vi "Open.vi"(8 "error in (no error)":errorcluster, 10 "Create if not exists? (T)":bool=TRUE, 11 "Path":path) -> (0 "error out":errorcluster, 1 "File Exists?":bool, 2 "File Created?":bool, 3 "LabVIEW-Config.lvlib:LabVIEW-Config.lvclass":refnum<class "LabVIEW-Config.lvclass">)   [LabVIEW 2017, in "LabVIEW-Config.lvlib" / "LabVIEW-Config.lvclass"]
uses:
  LabVIEW-Config.lvclass
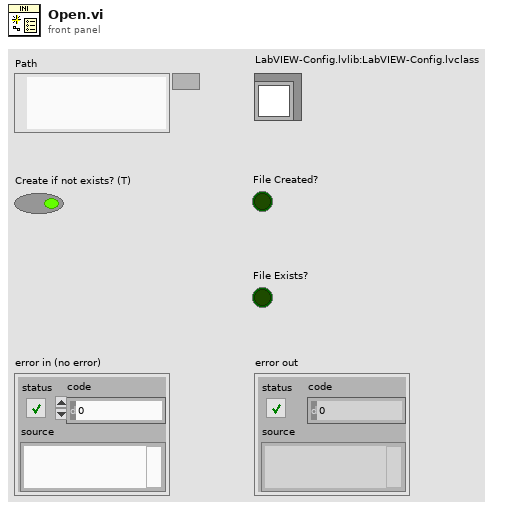
[diagram p1: front panel]
types:
  T1 = enum16{"open", "replace", "create", "open or create", "replace or create", "replace or create with confirmation"}
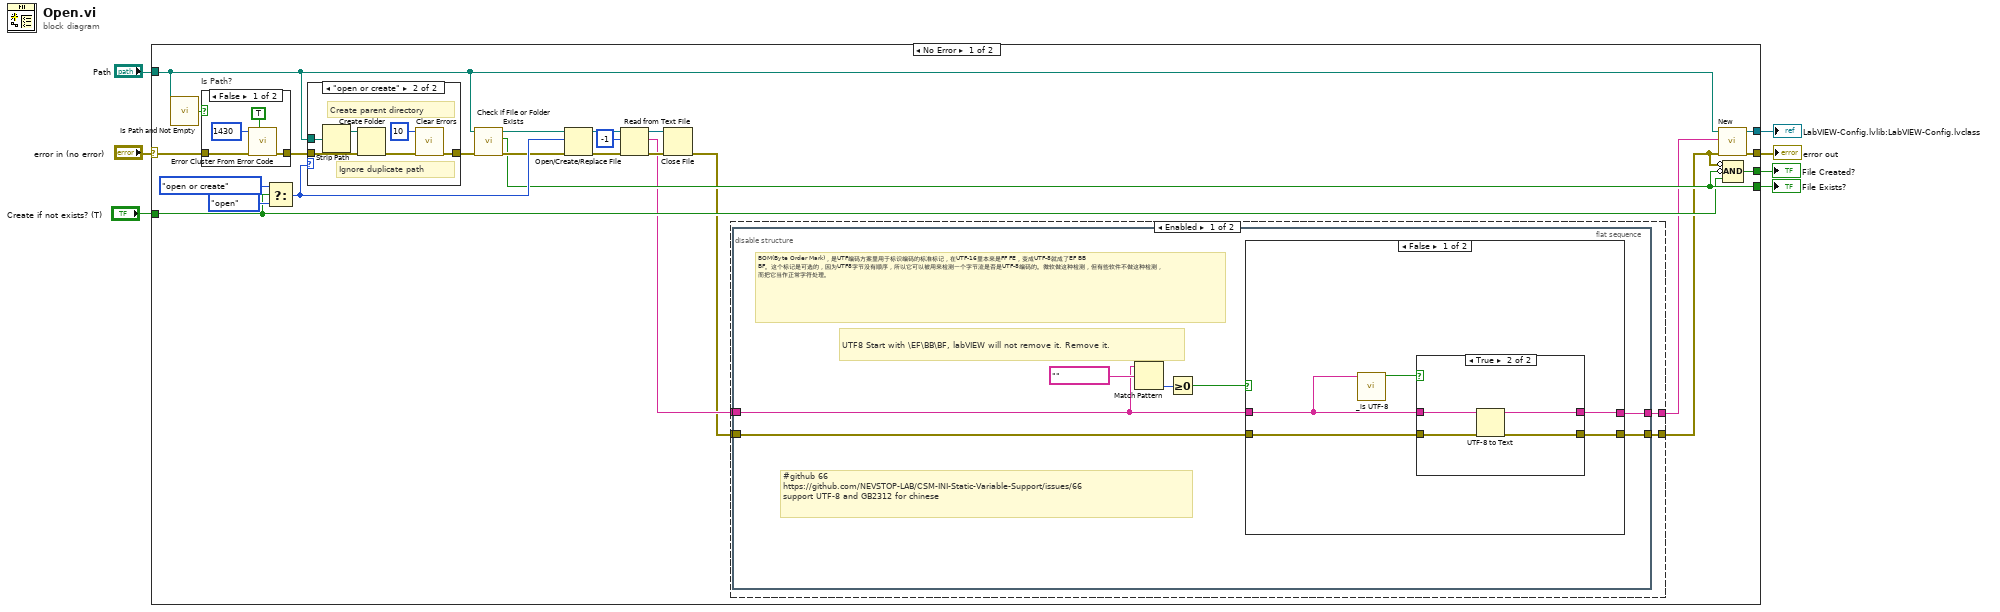
[diagram p0: block diagram]
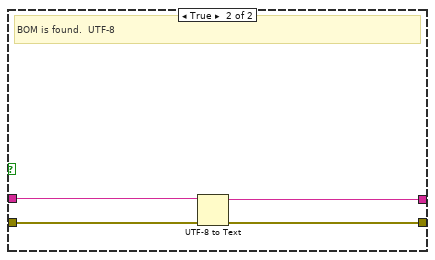
[diagram p3: hidden frame]
diagram:
  n1 = case shown="No Error" "error in (no error)" {
    selector: "error in (no error)" -> [w26 w72]
    tunnel: [w13 _] -> w7
    tunnel: [w15 w72] -> w5
    tunnel: "Create if not exists? (T)" -> [w12 _]
    tunnel: "Path" -> [w14 _]
    tunnel: [w17 _] -> w2
    tunnel: [w16 _] -> w1
    frame No Error {
      n2 = call <vilib>:"Is Path and Not Empty.vi"("path"=w14) -> ("Is Path and Not Empty?"=w20:bool)  [unwired: 4 in]
      n3 = case "Is Path?" shown="False" w20 {
        tunnel: w26 -> [w63 w64]
        tunnel: [w61 w64] -> w23
        frame False {
          n4 = call <vilib>:"Error Cluster From Error Code.vi"("show call chain? (False)"=TRUE, "error in (no error)"=w63, "error code (0)"=1430) -> ("error out"=w61:errorcluster)  [unwired: 6 in]
        }
        frame True {
        }
      }
      n5 = Select(t=T1."open or create" ("operation (0:open)"), s=w12, f=T1."open" ("operation (0:open)")) -> (s? t:f=w21:T1)
      n6 = case shown="\"open or create\"" w21 {
        tunnel: w23 -> [w65 w71]
        tunnel: [w65 w66] -> w22
        tunnel: w14 -> [_ w70]
        frame Default {
        }
        frame "open or create" {
          # "Create parent directory"
          # "Ignore duplicate path"
          n7 = Strip Path(path=w70) -> (stripped path=w69:path)  [unwired: 1 out]
          n8 = Create Folder(path (use dialog)=w69, error in=w71) -> (error out=w67:errorcluster)  [unwired: 1 in, 2 out]
          n9 = call <vilib>:"Clear Errors.vi"("error in (no error)"=w67, "specific error code to clear (0: all)"=10 ("Not Found")) -> ("error out"=w66:errorcluster)  [unwired: 4 in, 1 out]
        }
      }
      n10 = call <vilib>:"Check if File or Folder Exists.vi"("error in (no error)"=w22, "path"=w14) -> ("error out"=w19:errorcluster, "file or folder exists?"=w17:bool, "dup path"=w18:path)  [unwired: 7 in]
      n11 = Open/Create/Replace File(file path (use dialog)=w18, error in=w19, operation (0:open)=w21) -> (refnum out=w28:refnum<file>, error out=w29:errorcluster)  [unwired: 3 in, 1 out]
      n12 = Read from Text File(file (use dialog)=w28, count=-1, error in=w29) -> (refnum out=w30:refnum<file>, text=w11:string, error out=w31:errorcluster)  [unwired: 1 in, 1 out]
      n13 = Close File(refnum=w30, error in=w31) -> (error out=w10:errorcluster)  [unwired: 1 out]
      n14 = disable-structure shown="Enabled" {
        disable-tunnel: w11 -> [w35 w59]
        disable-tunnel: w10 -> [w34 w58]
        disable-tunnel: [w33 w58] -> w9
        disable-tunnel: [w32 w59] -> w8
        frame Enabled {
          n15 = flat-sequence {
            tunnel: w35 -> [w39]
            tunnel: w34 -> [w38]
            tunnel: [w37] -> w33
            tunnel: [w36] -> w32
            frame #0 {
              # "#github 66\nhttps://github.com/NEVSTOP-LAB/CSM-INI-Static-Variable-Support/issues/66\nsupport UTF-8 and GB2312 for chinese"
              # "BOM(Byte Order Mark)，是UTF编码方案里用于标识编码的标准标记，在UTF-16里本来是FF FE，变成UTF-8就成了EF BB BF。这个标记是可选的，因为UTF8字节没有顺序，所以它可以被用来检测一个字节流是否是UTF-8编码的。微软做这种检测，但有些软件不做这种检测， 而把它当作正常字符处理。"
              # "UTF8 Start with \\EF\\BB\\BF, labVIEW will not remove it. Remove it."
              n16 = Match Pattern(string=w39, regular expression="﻿") -> (offset past match=w41:i32)  [unwired: 1 in, 3 out]
              n17 = Greater Or Equal To 0?(x=w41) -> (x >= 0?=w42:bool)
              n18 = case shown="False" w42 {
                tunnel: [w46 w56] -> w36
                tunnel: w39 -> [w45 w57]
                tunnel: w38 -> [w43 w55]
                tunnel: [w44 w54] -> w37
                frame False {
                  n19 = call "_is UTF-8.vi"("String"=w45) -> ("UTF8"=w47:bool)  [unwired: 10 in]
                  n20 = case shown="True" w47 {
                    tunnel: w45 -> [w48 w53]
                    tunnel: [w48 w52] -> w46
                    tunnel: w43 -> [w49 w51]
                    tunnel: [w49 w50] -> w44
                    frame False {
                    }
                    frame True {
                      n21 = UTF-8 to Text(8:w51, 11:w53) -> (0:w50:errorcluster, 3:w52:string)  [unwired: 1 in]
                    }
                  }
                }
                frame True {
                  # "BOM is found.  UTF-8"
                  n22 = UTF-8 to Text(8:w55, 11:w57) -> (0:w54:errorcluster, 3:w56:string)  [unwired: 1 in]
                }
              }
            }
          }
        }
        frame Disabled {
        }
      }
      n23 = call "New.vi"("error in (no error)"=w9, "Text"=w8, "Path (\"\")"=w14) -> ("error out"=w15:errorcluster, "LabVIEW-Config.lvlib:LabVIEW-Config.lvclass"=w13:refnum<class "LabVIEW-Config.lvclass">)  [unwired: 7 in]
      n24 = Compound Arithmetic op=AND(invert w9, invert w17, w12) -> (w16:bool)
    }
    frame Error {
    }
  }
  "error out" <- w5
  "LabVIEW-Config.lvlib:LabVIEW-Config.lvclass" <- w7
  "File Exists?" <- w2
  "File Created?" <- w1
